vi "Experiment header-bundle and save.vi"(8 "error in (no error)":errorcluster, 10 "AOL_Globals":T1={"Imaging Protocol"=enum."AOL Z-Stack", "Number of POI"=0, "Number of Miniscans"=0, "Number of Trials"=0, "Number of Cycles "=0, "# Averaged Frames"=0, "Laser power (%)"=0, "Pockels (V)"=0.0, "Acquisition Length (sec)"=0.0, "Fill time (us)"=0.0, "POI Dwell time (us)"=0.0, "Miniscan Dwell time per pixel (us)"=0.0, "PMT 1"=0.0, "PMT 2"=0.0, "Back Apperture (mA)"=200.0, "Frame Size"=0, "Center Frequency"=0.0, "Field of View (norm)"=0.0, "DwellTime (us)"=0.0, "Wavelength (nm)"=0.0, "Zoom"=0.0, "AOL Z"=0.0, "AOL Mode"=enum."Raster", "GridXY"=0.0, "GridZ"=0.0, "TriggerPeriod (sec)"=0.0, "Number of Pixels in Miniscan"=0, "Experiment folder path"=path "", "X centre"=0.0, "Y centre"=0.0, "Angle (degrees)"=0.0, "Plane Mode"=0, "Threshold"=[], "Regenerate Chirps"=FALSE, "Rectangle ROI length (pixels)"=0, "Rectangle ROI height (pixels)"=0, "AOD fill"=4900, "StartupDelay"=0, "Samples Wait after Trigger"=5080, "Slip Cycle"=600000, "Add Cycle"=TRUE, "Functional Mode"=enum."Point", "Z Start"=0.0, "Z Stop"=0.0, "# Planes"=0} {"Plane Mode" items=["XY Plane", "XZ Plane", "YZ Plane", "arbitraryplane"]; "Frame Size" items=["100X100"=100, "128X128"=128, "200X200"=200, "256X256"=256, "512X512"=512, "1024x1024"=1024, "2048x2048"=2048]; "Back Apperture (mA)" format="%#.6g"; "Pockels (V)" format="%#.6g"; "PMT 2" format="%#.6g"; "PMT 1" format="%#.6g"; "Angle (degrees)" format="%#.6g"; "POI Dwell time (us)" format="%#.6g"}, 11 "Experiment data folder path":path) -> (0 "error out":errorcluster)   [LabVIEW 2017]
uses:
  Typedefs/Controls/AOL_Globals.ctl
  Typedefs/Imaging Protocols enum.ctl
  Typedefs/Frame Size.ctl
  Typedefs/AOL modes.ctl
  Typedefs/Plane Mode.ctl
  Typedefs/Functional Mode.ctl
  Typedefs/Header file interface module functions enum.ctl
  Typedefs/Header file sections.ctl
  Typedefs/Header file type enum.ctl
panel:
  out "Parameter Index":i32[](array[numeric])
  out "Parameter Value":dbl[](array[numeric])
  out "Parameter Name":string[](array[string])
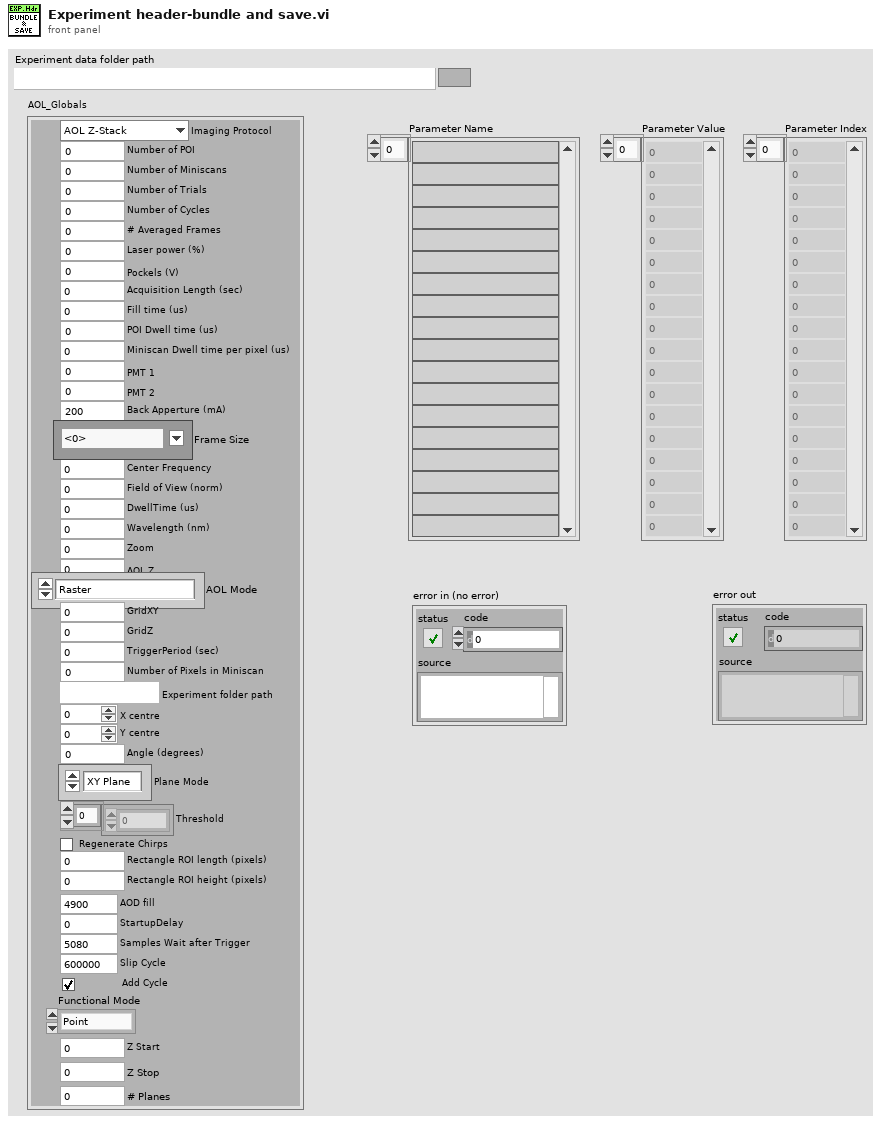
[diagram p1: front panel]
types:
  T1 = typedef "AOL_Globals.ctl" = cluster{"Imaging Protocol":T2, "Number of POI":u16, "Number of Miniscans":u16, "Number of Trials":u16, "Number of Cycles ":u64, "# Averaged Frames":u16, "Laser power (%)":u8, "Pockels (V)":dbl, "Acquisition Length (sec)":dbl, "Fill time (us)":dbl, "POI Dwell time (us)":dbl, "Miniscan Dwell time per pixel (us)":dbl, "PMT 1":dbl, "PMT 2":dbl, "Back Apperture (mA)":dbl, "Frame Size":T3, "Center Frequency":dbl, "Field of View (norm)":dbl, "DwellTime (us)":dbl, "Wavelength (nm)":dbl, "Zoom":dbl, "AOL Z":dbl, "AOL Mode":T4, "GridXY":dbl, "GridZ":dbl, "TriggerPeriod (sec)":dbl, "Number of Pixels in Miniscan":u16, "Experiment folder path":path, "X centre":dbl, "Y centre":dbl, "Angle (degrees)":dbl, "Plane Mode":T5, "Threshold":u16[], "Regenerate Chirps":bool, "Rectangle ROI length (pixels)":u16, "Rectangle ROI height (pixels)":u16, "AOD fill":u16, "StartupDelay":i32, "Samples Wait after Trigger":u16, "Slip Cycle":u32, "Add Cycle":bool, "Functional Mode":T6, "Z Start":dbl, "Z Stop":dbl, "# Planes":i32}
  T2 = typedef "Imaging Protocols enum.ctl" = enum16{"AOL Z-Stack", "Motor Z Stack", "Functional Acquisition", "Single Plane Acquisition", "Volume Acquisition", "Live Imaging", "Live Plane Imaging", "Live Volume Imaging"}
  T3 = typedef "Frame Size.ctl" = u16
  T4 = typedef "AOL modes.ctl" = enum16{"Raster", "Structural", "Pointing", "Mini Scan", "Alignment"}
  T5 = typedef "Plane Mode.ctl" = u16
  T6 = typedef "Functional Mode.ctl" = enum16{"Point", "Line", "Patch", "Plane", "Volume"}
  T7 = typedef "Header file type enum.ctl" = enum16{"All parameters", "Params for funct acq w ROI or mscn", "Params for funct acq w rectangles", "Live imaging header parameters", "AOL Parameters"}
  T8 = typedef "Header file sections.ctl" = enum16{"ALL SECTIONS", "LOGIN", "GLOBAL PARAMETERS", "IMAGING MODES", "TIME SERIES", "MOTOR Z-STACK", "AOL Z-STACK", "FUNCTIONAL IMAGING", "VOLUME IMAGING", "MOVEMENT CORRECTION", "CALIBRATION", "STATISTICS", "BIOLOGY INFORMATION"}
  T9 = typedef "Header file interface module functions enum.ctl" = enum16{"Load experiment header file", "Save experiment header file", "Clear stored values", "Read stored values", "Update specific value in memory", "Update values in memory"}
  T10 = typedef "Header file type enum.ctl" = enum16{"All parameters", "Login", "Global Parameters", "Imaging Modes", "Time Series", "Motor Zstack", "AOL Zstack", "Functional Imaging", "Movement Correction", "Calibration Setup", "Statistics", "Biology Information"}
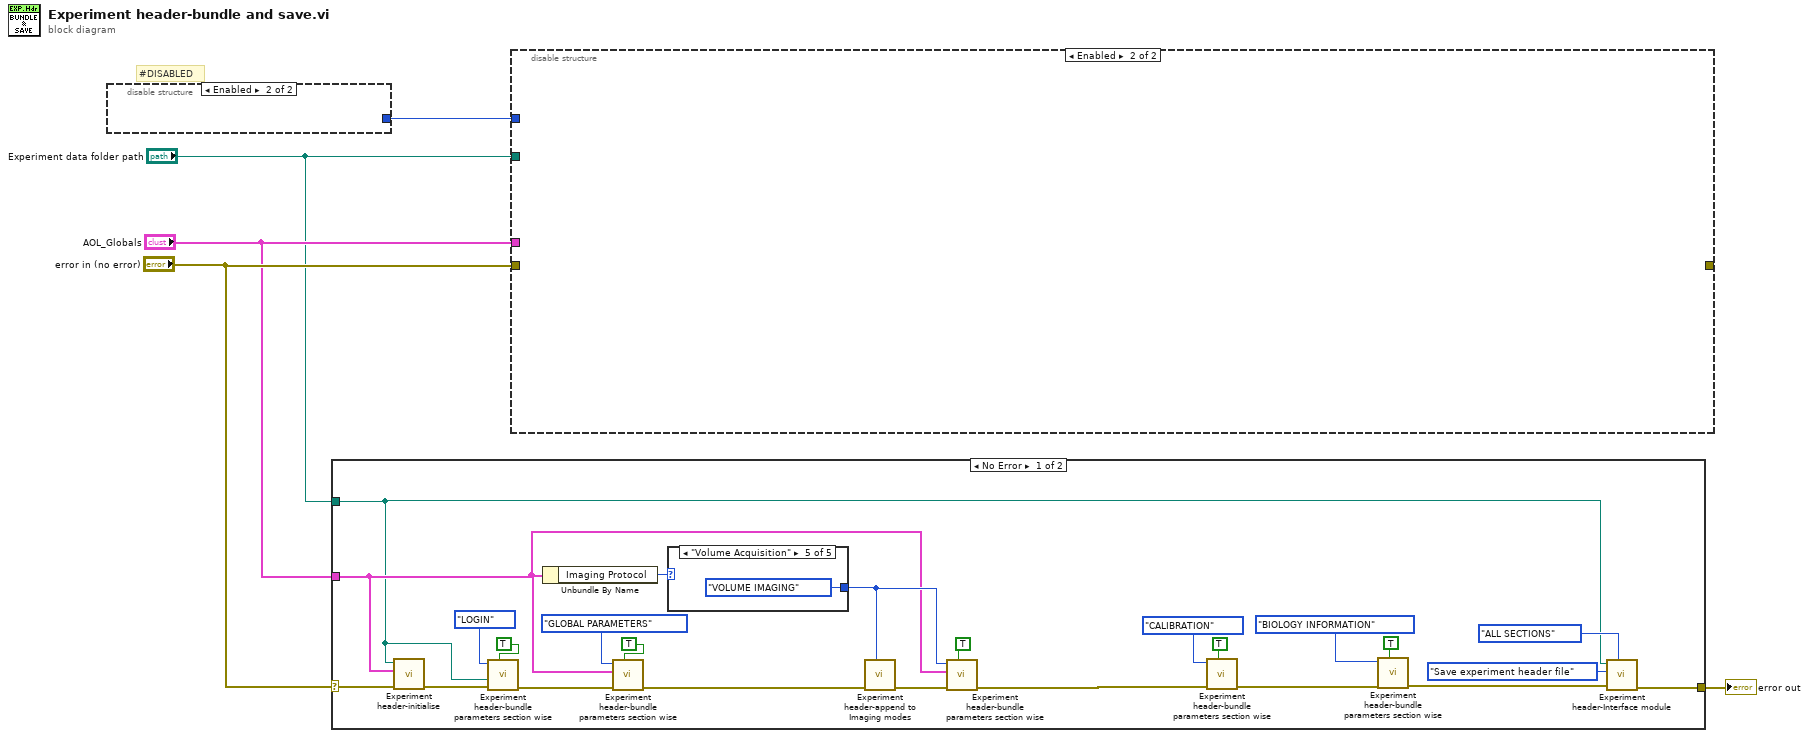
[diagram p0: block diagram]
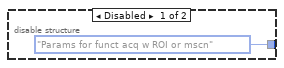
[diagram p2: hidden frame]
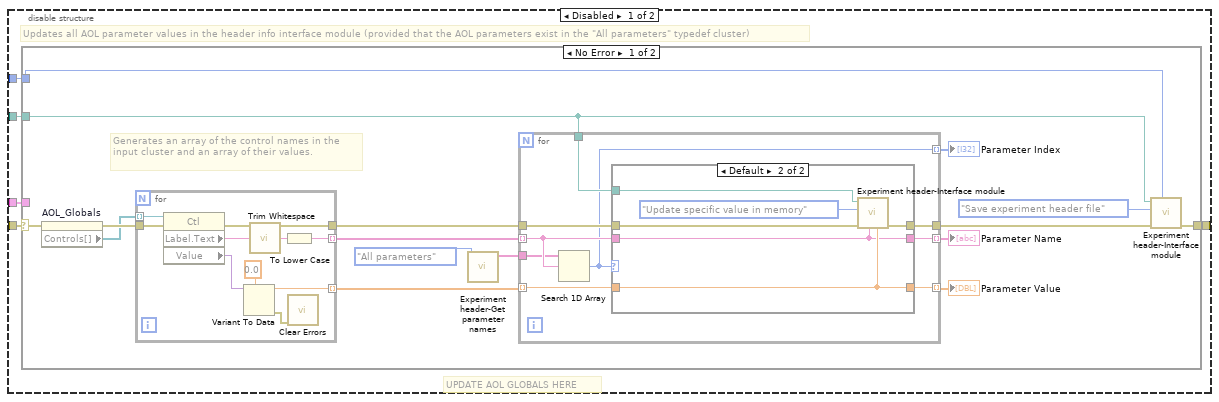
[diagram p3: hidden frame]
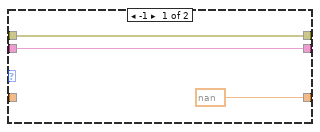
[diagram p4: hidden frame]
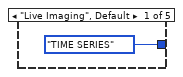
[diagram p6: hidden frame]
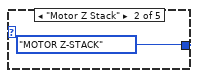
[diagram p7: hidden frame]
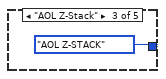
[diagram p8: hidden frame]
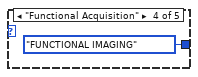
[diagram p9: hidden frame]
diagram:
  # "#DISABLED"
  n1 = disable-structure shown="Enabled" {
    disable-tunnel: [Header_file_type_enum."Params for funct acq w ROI or mscn" ("Header file type") _] -> w5
    frame Disabled {
    }
    frame Enabled {
    }
  }
  n2 = case shown="No Error" "error in (no error)" {
    selector: "error in (no error)" -> [w25 w36]
    tunnel: "AOL_Globals" -> [w18 _]
    tunnel: [w29 w36] -> w2
    tunnel: "Experiment data folder path" -> [w8 _]
    frame No Error {
      n3 = call "Experiment header-initialise.vi"("error in (no error)"=w25, "AOL_Globals"=w18, "Experiment data folder path"=w8) -> ("error out"=w22:errorcluster)  [unwired: 8 in]
      n4 = call "Experiment header-bundle parameters section wise.vi"("Update header\ninterface cluster ?"=TRUE ("Update header\ninterface cluster ?"), "error in (no error)"=w22, "Experiment data folder path"=w8, "Header file sections"=Header_file_sections."LOGIN") -> ("error out"=w17:errorcluster)  [unwired: 6 in, 1 out]
      n5 = Unbundle By Name(w18) -> ("Imaging Protocol"=w30:T2)
      n6 = call "Experiment header-bundle parameters section wise.vi"("Update header\ninterface cluster ?"=TRUE ("Update header\ninterface cluster ?"), "error in (no error)"=w17, "AOL_Globals"=w18, "Header file sections"=Header_file_sections."GLOBAL PARAMETERS") -> ("error out"=w16:errorcluster)  [unwired: 6 in, 1 out]
      n7 = case shown="\"Volume Acquisition\"" w30 {
        tunnel: [Header_file_sections."TIME SERIES" ("Header file sections") Header_file_sections."MOTOR Z-STACK" ("Header file sections") Header_file_sections."AOL Z-STACK" ("Header file sections") Header_file_sections."FUNCTIONAL IMAGING" ("Header file sections") Header_file_sections."VOLUME IMAGING" ("Header file sections")] -> w26
        frame "Live Imaging", Default {
        }
        frame "Motor Z Stack" {
        }
        frame "AOL Z-Stack" {
        }
        frame "Functional Acquisition" {
        }
        frame "Volume Acquisition" {
        }
      }
      n8 = call "Experiment header-append to Imaging modes.vi"("Header file sections"=w26, "error in (no error)"=w16) -> ("error out"=w27:errorcluster)  [unwired: 9 in]
      n9 = call "Experiment header-bundle parameters section wise.vi"("Update header\ninterface cluster ?"=TRUE ("Update header\ninterface cluster ?"), "error in (no error)"=w27, "AOL_Globals"=w18, "Header file sections"=w26) -> ("error out"=w7:errorcluster)  [unwired: 6 in, 1 out]
      n10 = call "Experiment header-bundle parameters section wise.vi"("Update header\ninterface cluster ?"=TRUE ("Update header\ninterface cluster ?"), "error in (no error)"=w7, "Header file sections"=Header_file_sections."CALIBRATION") -> ("error out"=w11:errorcluster)  [unwired: 7 in, 1 out]
      n11 = call "Experiment header-bundle parameters section wise.vi"("Update header\ninterface cluster ?"=TRUE ("Update header\ninterface cluster ?"), "error in (no error)"=w11, "Header file sections"=Header_file_sections."BIOLOGY INFORMATION") -> ("error out"=w10:errorcluster)  [unwired: 7 in, 1 out]
      n12 = call "Experiment header-Interface module.vi"("Header file sections"=Header_file_sections."ALL SECTIONS", "error in (no error)"=w10, "Function"=Header_file_interface_module_functions_enum."Save experiment header file", "Experiment data folder path"=w8) -> ("error out"=w29:errorcluster)  [unwired: 6 in, 1 out]
    }
    frame Error {
    }
  }
  "error out" <- w2
  n13 = disable-structure shown="Enabled" {
    disable-tunnel: [w41 _] -> _
    disable-tunnel: w5 -> [w40 _]
    disable-tunnel: "Experiment data folder path" -> [w39 _]
    disable-tunnel: "error in (no error)" -> [w38 _]
    disable-tunnel: "AOL_Globals" -> [w37 _]
    frame Disabled {
      # "UPDATE AOL GLOBALS HERE"
      # "Updates all AOL parameter values in the header info interface module (provided that the AOL parameters exist in the \"All parameters\" typedef cluster)"
      n14 = case shown="No Error" w38 {
        selector: w38 -> [w55 w86]
        tunnel: [w57 w86] -> w41
        tunnel: w39 -> [w56 _]
        tunnel: w37 -> [_ _]
        tunnel: w40 -> [w42 _]
        frame No Error {
          # "Generates an array of the control names in the input cluster and an array of their values."
          n15 = property on="AOL_Globals" class="Clust (strict)"(error in=w55) -> (error out=w51:errorcluster, "Controls[]"=w47:refnum<vi>[])  [unwired: 1 in, 1 out]
          n16 = for {
            tunnel: [w83] -> w53 mode=indexing
            tunnel: w47 -> [w80] mode=indexing
            tunnel: w51 -> [w82]
            tunnel: [w79] -> w44
            tunnel: [w76] -> w43 mode=indexing
            n17 = property class="Ctl"(reference=w80, error in=w82) -> (error out=w79:errorcluster, "Label.Text"=w77:string, "Value"=w85:variant)  [unwired: 1 out]
            n18 = Variant To Data(type=0.0, Variant=w85) -> (data=w83:dbl, error out=w81:errorcluster)  [unwired: 1 in]
            n19 = call <vilib>:"Trim Whitespace.vi"("string"=w77) -> ("trimmed string"=w78:string)  [unwired: 1 in]
            n20 = To Lower Case(string=w78) -> (all lower case string=w76:string)
            n21 = call <vilib>:"Clear Errors.vi"("error in (no error)"=w81) -> ()  [unwired: 5 in, 2 out]
          }
          n22 = call "Experiment header-Get parameter names.vi"("Section Refs"=Header_file_type_enum."All parameters" ("Header file type")) -> ("Section Names"=w45:string[])  [unwired: 8 in, 2 out]
          n23 = for {
            tunnel: w43 -> [w60] mode=indexing
            tunnel: [w66] -> w54 mode=indexing
            tunnel: w53 -> [w65] mode=indexing
            tunnel: [w64] -> w52 mode=indexing
            tunnel: [w62] -> w49
            tunnel: w44 -> [w63]
            tunnel: w56 -> [w61]
            tunnel: [w59] -> w48 mode=indexing
            tunnel: w45 -> [w58]
            n24 = Search 1D Array(1D array=w58, element=w60) -> (index of element=w59:i32)  [unwired: 1 in]
            n25 = case shown="Default" w59 {
              tunnel: [w67 w71] -> w66
              tunnel: w65 -> [_ w72]
              tunnel: [nan w72] -> w64
              tunnel: w63 -> [w69 w70]
              tunnel: [w69 w74] -> w62
              tunnel: w61 -> [_ w73]
              tunnel: w60 -> [w67 w71]
              frame -1 {
              }
              frame Default {
                n26 = call "Experiment header-Interface module.vi"("Value to change"=w72, "Name of parameter to update"=w71, "error in (no error)"=w70, "Function"=Header_file_interface_module_functions_enum."Update specific value in memory", "Experiment data folder path"=w73) -> ("error out"=w74:errorcluster)  [unwired: 5 in, 1 out]
              }
            }
          }
          "Parameter Name" <- w54
          "Parameter Value" <- w52
          "Parameter Index" <- w48
          n27 = call "Experiment header-Interface module.vi"("Header file sections"=w42, "error in (no error)"=w49, "Function"=Header_file_interface_module_functions_enum."Save experiment header file", "Experiment data folder path"=w56) -> ("error out"=w57:errorcluster)  [unwired: 6 in, 1 out]
        }
        frame Error {
        }
      }
    }
    frame Enabled {
    }
  }
